vi "Ctor.vi"(8 "error in (no error)":errorcluster) -> (0 "error out":errorcluster, 3 "LV Chat Server out":refnum<class "LV Chat Server.lvclass">)   [LabVIEW 2020, in "LV Chat Server.lvclass"]
uses:
  LV Chat Server.lvclass
  Ref Data.ctl
  User.ctl
  Stream-Simple-Msg/Endpoint/Endpoint.lvclass
  LV Chat Server.lvclass/LV Chat Server.ctl
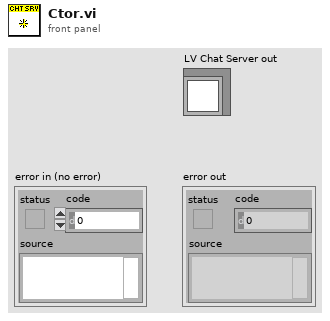
[diagram p1: front panel]
types:
  T1 = typedef "LV Chat Server.lvclass/Ref Data.ctl" = cluster{"User Map":map{string, T2}}
  T2 = typedef "LV Chat Server.lvclass/User.ctl" = cluster{"Name":string, "IP":string, "Connected At":dbl, "Endpoint":refnum<class "Endpoint.lvclass">}
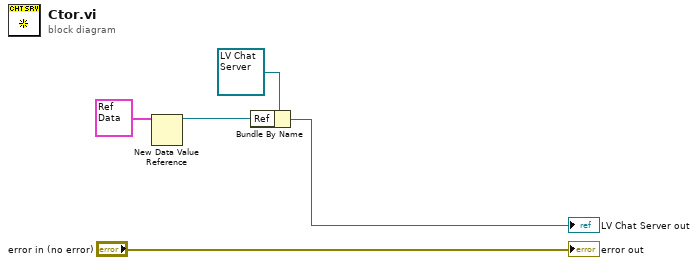
[diagram p0: block diagram]
diagram:
  n1 = New Data Value Reference(data value=T1 {"User Map"={}} ("Ref Data")) -> (data value reference=w1:refnum<data-value>)  [unwired: 1 in, 1 out]
  n2 = Bundle By Name(cluster=refnum<class "LV Chat Server.lvclass"> refnum ("LV Chat Server in"), "Ref"=w1) -> (→"LV Chat Server out":refnum<class "LV Chat Server.lvclass">)
  "error out" <- "error in (no error)"
